vi "RT Web Variables.vi"() -> ()   [LabVIEW 2014]
panel:
  out "VariableIndicator 2":dbl
  in  "Stop":bool
  out "VariableIndicator":dbl
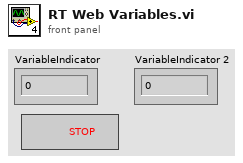
[diagram p1: front panel]
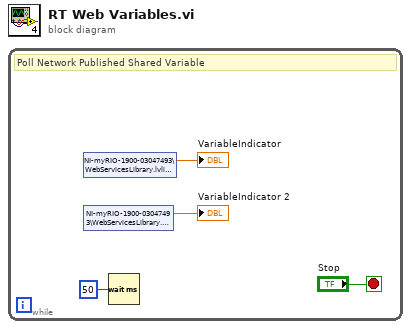
[diagram p0: block diagram]
diagram:
  n1 = while {
    stop <- "Stop" stop-if-true
    # "Poll Network Published Shared Variable"
    n2 = shared-variable "NI-myRIO-1900-03047493\\WebServicesLibrary.lvlib\\Direction"() -> (→"VariableIndicator":dbl)  [unwired: 1 in, 1 out]
    n3 = shared-variable "NI-myRIO-1900-03047493\\WebServicesLibrary.lvlib\\Connect"() -> (→"VariableIndicator 2":dbl)  [unwired: 1 in, 1 out]
    n4 = Wait (ms)(milliseconds to wait=u32 50) -> ()  [unwired: 1 out]
  }
